vi "MonochromatorOffsets.vi"(7 "Operation":T1, 8 "error in (no error)":errorcluster, 11 "offsetsIn":string[][](array[string])) -> (0 "error out":errorcluster, 1 "Channel":string[](array[string]), 2 "offsets":dbl[](array[numeric]), 3 "offsets Out":string[][](array[string]))   [LabVIEW 2018]
uses:
  Strict Type Controls/Settings Operation.ctl
  <vilib>/Utility/file.llb/Read From Spreadsheet File (string).vi
  <vilib>/Utility/file.llb/Write To Spreadsheet File (string).vi
panel:
  # "N1\t93,81\nN2\t157,81\nN3\t92,114\nN4\t157,80"
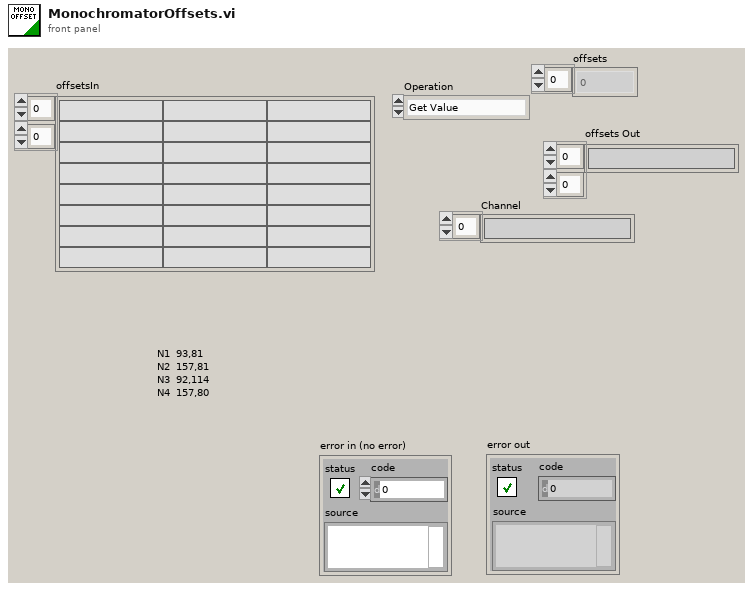
[diagram p1: front panel]
types:
  T1 = typedef "Settings Operation.ctl" = enum8{"Get Value", "Set Value", "Read File", "Write File", "Write Stored Value"}
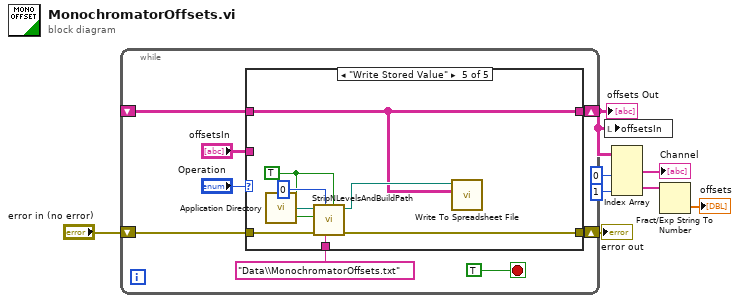
[diagram p0: block diagram]
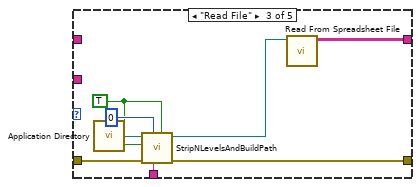
[diagram p4: hidden frame]
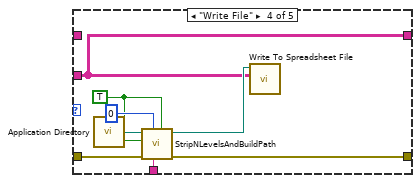
[diagram p5: hidden frame]
diagram:
  n1 = while {
    shift-right: [w15] -> w6
    shift-left: _ -> [w16]
    shift-right: [w12] -> w7
    shift-left: "error in (no error)" -> [w13]
    stop <- TRUE stop-if-true
    n2 = case shown="\"Write Stored Value\"" "Operation" {
      tunnel: w16 -> [w18 _ _ _ w38]
      tunnel: [w18 w20 w22 w30 w38] -> w15
      tunnel: "offsetsIn" -> [_ w20 _ w30 _]
      tunnel: w13 -> [w17 w19 w25 w35 w41]
      tunnel: [w17 w19 w21 w29 w37] -> w12
      tunnel: "Data\\MonochromatorOffsets.txt" ("Build Path") -> [_ _ w24 w32 w40]
      frame "Get Value" {
      }
      frame "Set Value" {
      }
      frame "Read File" {
        w26 = TRUE ("Is File?")
        n3 = call <vilib>:"Application Directory.vi"() -> ("Application Directory"=w28:path)
        n4 = call "StripNLevelsAndBuildPath.vi"("Create Folders"=w26, "Build Path"=w24, "Strip Levels"=0, "error in(no error)"=w25, "Is File"=w26, "Path In"=w28) -> ("error out"=w21:errorcluster, "Path Out"=w23:path)  [unwired: 4 out]
        n5 = call-poly <vilib>:"Read From Spreadsheet File.vi"("file path (dialog if empty)"=w23) -> ("all rows"=w22:string[][])  [unwired: 6 in, 4 out]
      }
      frame "Write File" {
        w33 = TRUE ("Is File?")
        n6 = call <vilib>:"Application Directory.vi"() -> ("Application Directory"=w36:path)
        n7 = call "StripNLevelsAndBuildPath.vi"("Create Folders"=w33, "Build Path"=w32, "Strip Levels"=0, "error in(no error)"=w35, "Is File"=w33, "Path In"=w36) -> ("error out"=w29:errorcluster, "Path Out"=w31:path)  [unwired: 4 out]
        n8 = call-poly <vilib>:"Write To Spreadsheet File.vi"("2D data"=w30, "file path (dialog if empty)"=w31) -> ()  [unwired: 6 in, 1 out]
      }
      frame "Write Stored Value" {
        w42 = TRUE ("Is File?")
        n9 = call <vilib>:"Application Directory.vi"() -> ("Application Directory"=w44:path)
        n10 = call "StripNLevelsAndBuildPath.vi"("Create Folders"=w42, "Build Path"=w40, "Strip Levels"=0, "error in(no error)"=w41, "Is File"=w42, "Path In"=w44) -> ("error out"=w37:errorcluster, "Path Out"=w39:path)  [unwired: 4 out]
        n11 = call-poly <vilib>:"Write To Spreadsheet File.vi"("2D data"=w38, "file path (dialog if empty)"=w39) -> ()  [unwired: 6 in, 1 out]
      }
    }
  }
  "error out" <- w7
  "offsets Out" <- w6
  n12 = local write "offsetsIn"(w6) -> ()
  n13 = Index Array(array=w6, index (col) #1=0 ("disabled index (col)"), index (col) #2=1 ("index (col)")) -> (element #1=→"Channel":string[], element #2=w3:string[])  [unwired: 2 in]
  n14 = Fract/Exp String To Number(string=w3) -> (number=→"offsets":dbl[])  [unwired: 3 in, 1 out]
